vi "insert_GUI.vi"(8 "error in (no error)":errorcluster, 9 "Pane":refnum<vi>, 10 "VI path":path, 11 "component in":refnum<class "GenericToplevelComponent.lvclass">) -> (0 "error out":errorcluster, 3 "component out":refnum<class "GenericToplevelComponent.lvclass">)   [LabVIEW 2011, in "GenericToplevelComponent.lvclass"]
uses:
  GenericToplevelComponent.lvclass
  <vilib>/Utility/miscctls.llb/LVPointTypeDef.ctl
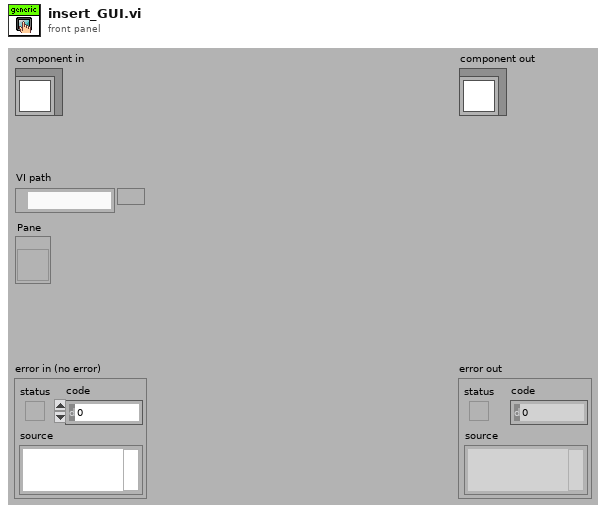
[diagram p1: front panel]
types:
  T1 = typedef "LVPointTypeDef.ctl" = cluster{"Horizontal":i16, "Vertical":i16}
  T2 = typedef "controls_refs.ctl" = cluster{"buttons":cluster{"start_focus":refnum<vi>, "start_single_sweep":refnum<vi>, "start_experiment":refnum<vi>, "save":refnum<vi>, "exit":refnum<vi>}, "tabs":cluster{"main":refnum<vi>, "settings":refnum<vi>}, "subpanels":cluster{"imagingMode":refnum<vi>, "scanHead":refnum<vi>, "display":refnum<vi>, "experimentController":refnum<vi>, "instrument":refnum<vi>, "stage":refnum<vi>, "stimulator":refnum<vi>, "dataCollection":refnum<vi>, "analyser":refnum<vi>, "daq":refnum<vi>, "imageAssembler":refnum<vi>}, "drop-downs":cluster{"imagingMode":refnum<vi>, "experimentalController":refnum<vi>, "objective":refnum<vi>}, "status lights":cluster{"experimentController":refnum<vi>, "imagingMode":refnum<vi>, "scanHead":refnum<vi>, "daq":refnum<vi>, "imageAssembler":refnum<vi>, "dataCollection":refnum<vi>, "display":refnum<vi>, "analyser":refnum<vi>, "stage":refnum<vi>, "stimulator":refnum<vi>, "instrument":refnum<vi>}, "message":refnum<vi>, "stimulator enabled?":refnum<vi>, "saving":cluster{"data folder path":refnum<vi>, "file base name":refnum<vi>, "notebook":refnum<vi>}, "progress bar":refnum<vi>, "update icon":refnum<vi>, "title":refnum<vi>, "main vi":refnum<vi>, "user":refnum<vi>}
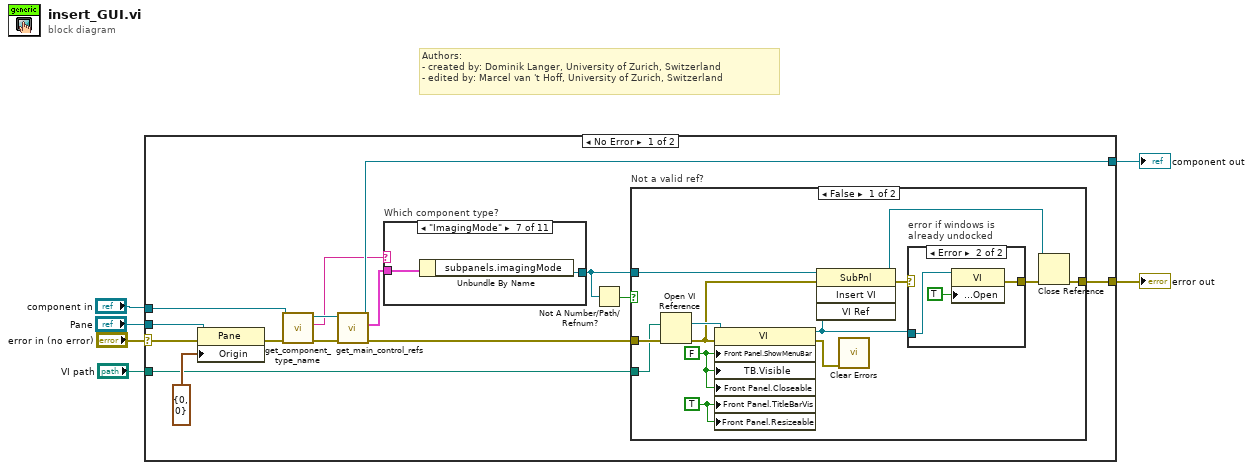
[diagram p0: block diagram]
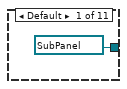
[diagram p4: hidden frame]
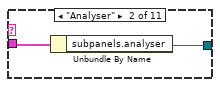
[diagram p5: hidden frame]
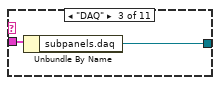
[diagram p6: hidden frame]
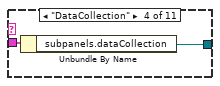
[diagram p7: hidden frame]
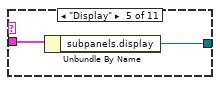
[diagram p8: hidden frame]
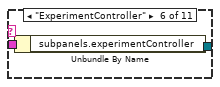
[diagram p9: hidden frame]
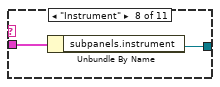
[diagram p10: hidden frame]
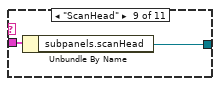
[diagram p11: hidden frame]
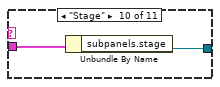
[diagram p12: hidden frame]
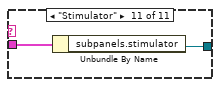
[diagram p13: hidden frame]
diagram:
  # "Authors: \n- created by: Dominik Langer, University of Zurich, Switzerland\n- edited by: Marcel van 't Hoff, University of Zurich, Switzerland"
  n1 = case shown="No Error" "error in (no error)" {
    selector: "error in (no error)" -> [w9 w62]
    tunnel: [w18 w62] -> w6
    tunnel: [w19 w61] -> w4
    tunnel: "component in" -> [w16 w61]
    tunnel: "VI path" -> [w7 _]
    tunnel: "Pane" -> [w10 _]
    frame No Error {
      n2 = property class="Pane"(reference=w10, error in=w9, "Origin"=T1 {"Horizontal"=0, "Vertical"=0}) -> (error out=w8:errorcluster)  [unwired: 1 out]
      n3 = call-dynamic "get_component_type_name.vi"("error in (no error)"=w8, "GenericPlugin in"=w16) -> ("error out"=w17:errorcluster, "component type"=w14:string, "GenericPlugin out"=w15:refnum<class "GenericToplevelComponent.lvclass">)  [unwired: 7 in]
      n4 = call-dynamic "get_main_control_refs.vi"("error in (no error)"=w17, "GenericPlugin.lvclass in"=w15) -> ("error out"=w21:errorcluster, "control references"=w20:T2, "GenericPlugin.lvclass out"=w19:refnum<class "GenericToplevelComponent.lvclass">)  [unwired: 7 out]
      n5 = case "Which component type?" shown="\"ImagingMode\"" w14 {
        tunnel: w20 -> [_ w42 w44 w45 w48 w50 w52 w54 w56 w58 w60]
        tunnel: [refnum<vi> refnum ("stimulator") w41 w43 w46 w47 w49 w51 w53 w55 w57 w59] -> w13
        frame Default {
        }
        frame "Analyser" {
          n6 = Unbundle By Name(w42) -> ("subpanels.analyser"=w41:refnum<vi>)
        }
        frame "DAQ" {
          n7 = Unbundle By Name(w44) -> ("subpanels.daq"=w43:refnum<vi>)
        }
        frame "DataCollection" {
          n8 = Unbundle By Name(w45) -> ("subpanels.dataCollection"=w46:refnum<vi>)
        }
        frame "Display" {
          n9 = Unbundle By Name(w48) -> ("subpanels.display"=w47:refnum<vi>)
        }
        frame "ExperimentController" {
          n10 = Unbundle By Name(w50) -> ("subpanels.experimentController"=w49:refnum<vi>)
        }
        frame "ImagingMode" {
          n11 = Unbundle By Name(w52) -> ("subpanels.imagingMode"=w51:refnum<vi>)
        }
        frame "Instrument" {
          n12 = Unbundle By Name(w54) -> ("subpanels.instrument"=w53:refnum<vi>)
        }
        frame "ScanHead" {
          n13 = Unbundle By Name(w56) -> ("subpanels.scanHead"=w55:refnum<vi>)
        }
        frame "Stage" {
          n14 = Unbundle By Name(w58) -> ("subpanels.stage"=w57:refnum<vi>)
        }
        frame "Stimulator" {
          n15 = Unbundle By Name(w60) -> ("subpanels.stimulator"=w59:refnum<vi>)
        }
      }
      n16 = Not A Number/Path/Refnum?(number/path/refnum=w13) -> (NaN/Path/Refnum?=w12:bool)
      n17 = case "Not a valid ref?" shown="False" w12 {
        tunnel: w21 -> [w34 w39]
        tunnel: [w30 w39] -> w18
        tunnel: w7 -> [w32 _]
        tunnel: w13 -> [w31 _]
        frame False {
          w29 = TRUE ("Front Panel Window:Title Bar Visible")
          w27 = FALSE ("Front Panel Window:Closeable")
          n18 = Open VI Reference(vi path=w32, error in (no error)=w34) -> (vi reference=w28:refnum<vi>, error out=w25:errorcluster)  [unwired: 1 in, 3 out]
          n19 = property class="VI"(reference=w28, error in=w25, "Front Panel.ShowMenuBar"=w27, "TB.Visible"=w27, "Front Panel.Closeable"=w27, "Front Panel.TitleBarVis"=w29, "Front Panel.Resizeable"=w29) -> (reference out=w22:refnum<vi>, error out=w26:errorcluster)
          n20 = invoke on="Invoke Node" class="SubPnl" method="Insert VI"(reference=w31, error in=w25, "VI Ref"=w22) -> (reference out=w33:refnum<vi>, error out=w24:errorcluster)  [unwired: 1 in, 2 out]
          n21 = call <vilib>:"Clear Errors.vi"("error in (no error)"=w26) -> ()  [unwired: 6 in, 1 out]
          n22 = case "error if windows is \nalready undocked" shown="Error" w24 {
            selector: w24 -> [w35 _]
            tunnel: [w35 w37] -> w23
            tunnel: w22 -> [_ w36]
            frame No Error {
            }
            frame Error {
              n23 = property class="VI"(reference=w36, "Front Panel.Open"=TRUE ("Front Panel Window:Open")) -> (error out=w37:errorcluster)  [unwired: 1 in, 1 out]
            }
          }
          n24 = Close Reference(reference=w33, error in (no error)=w23) -> (error out=w30:errorcluster)
        }
        frame True {
        }
      }
    }
    frame Error {
    }
  }
  "error out" <- w6
  "component out" <- w4
